vi "sParseRad7String.vi"(0 "Rad7 Input data":string="0501 2.69 \" 2.83 p Sniff\nFRI 21-MAY-99 19:41\n26.8 EC RH: 7% B:7.06V\nTotal Counts: 42.\nLivetime: 27.8min\nA: 0.53\"0.08 cpm 47.3%\nB: 0.02\"0.02 cpm 1.7%\nC: 0.52\"0.08 cpm 46.4%\nD: 0.01\"0.02 cpm 0.9%\nO: 0.04\"0.03 cpm 3.6%") -> (1 "Datanames":string[](array[string]), 2 "Data":dbl[](array[numeric]))   [LabVIEW 2012]
panel:
  out "substring before match":string
  out "array 2":string[][](array[string])
  out "Array":dbl[](array[numeric])
  out "appended array":string[](array[string])
  out "array":string[][](array[string])
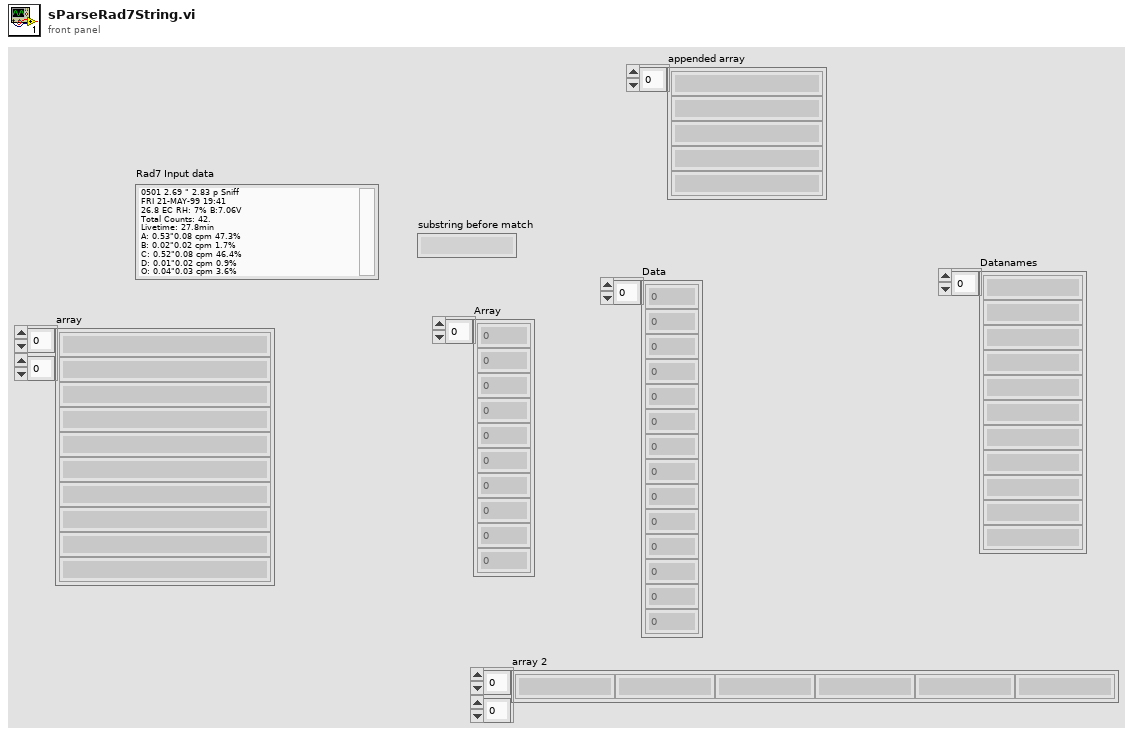
[diagram p1: front panel]
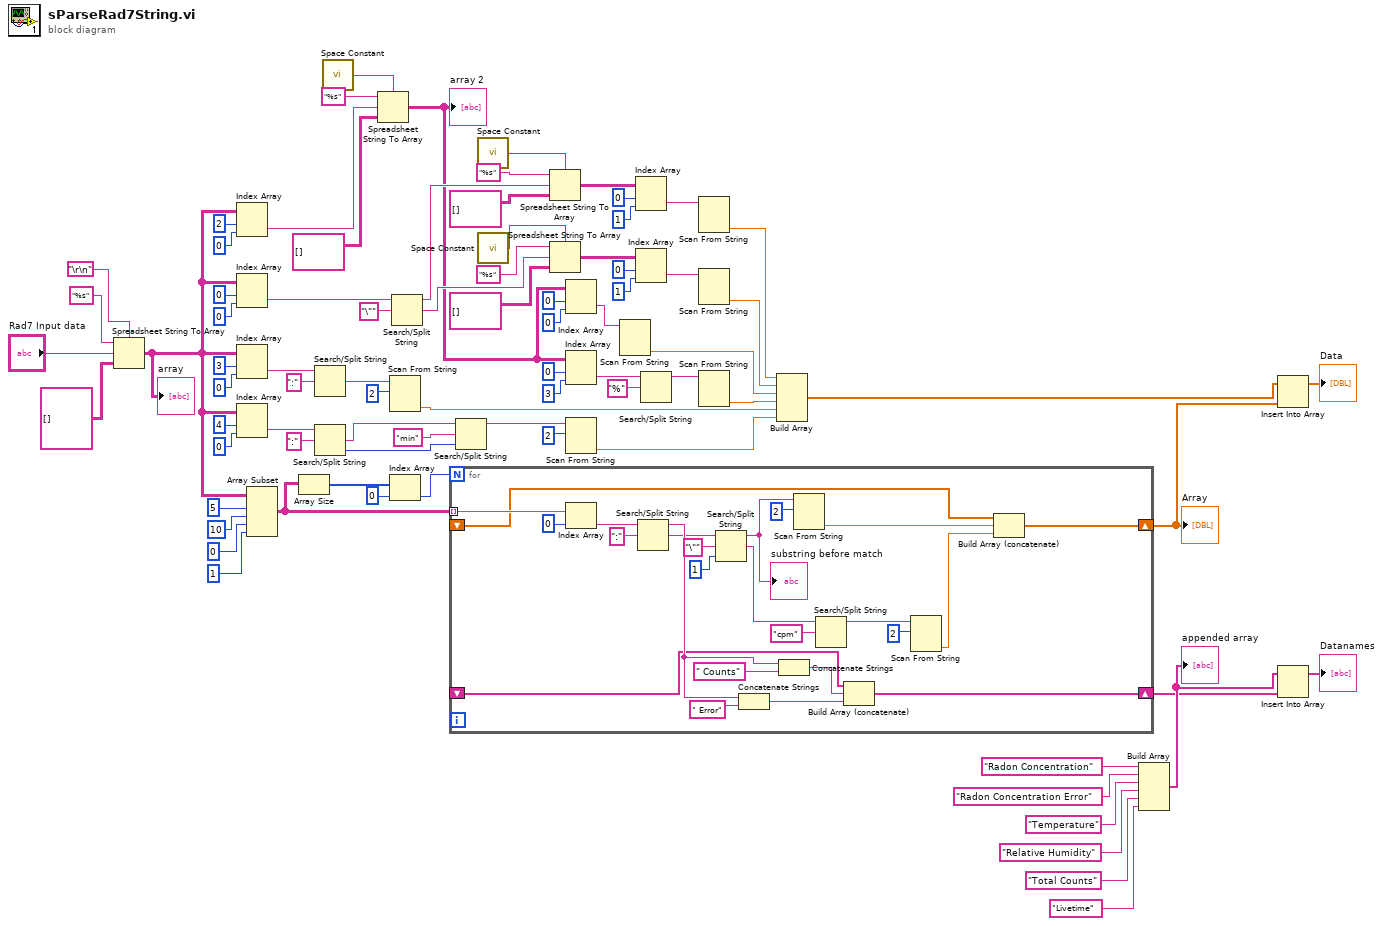
[diagram p0: block diagram]
diagram:
  n1 = Spreadsheet String To Array(delimiter (Tab)="\r\n", format string="%s", spreadsheet string="Rad7 Input data", array type (2D Dbl)=string[][] []) -> (array=w6:string[][])
  "array" <- w6
  n2 = Index Array(array=w6, index (row)=2, index (col)=0) -> (element=w39:string)
  n3 = Index Array(array=w6, index (row)=0, index (col)=0 ("disabled index (col)")) -> (element=w70:string)
  n4 = Index Array(array=w6, index (row)=3, index (col)=0) -> (element=w5:string)
  n5 = Index Array(array=w6, index (row)=4, index (col)=0) -> (element=w18:string)
  n6 = Array Subset(array=w6, index (row)=5 ("index"), length (row)=10 ("length"), index (col)=0 ("index"), length (col)=1 ("length")) -> (w48:string[][])
  n7 = Array Size(array=w48) -> (size(s)=w51:i32[])
  n8 = Search/Split String(string=w5, search string/char (-)=":") -> (match + rest of string=w3:string)  [unwired: 1 in, 2 out]
  n9 = Search/Split String(string=w18, search string/char (-)=":") -> (match + rest of string=w16:string, offset of match=w14:i32)  [unwired: 1 in, 1 out]
  n10 = call <vilib>:"Space Constant.vi"() -> ("String"=w42:string)
  n11 = Spreadsheet String To Array(delimiter (Tab)=w42, format string="%s", spreadsheet string=w39, array type (2D Dbl)=string[][] []) -> (array=w23:string[][])
  "array 2" <- w23
  n12 = Scan From String(input string=w3, initial scan location=u32 2) -> (output 1=w1:dbl)  [unwired: 3 in, 3 out]
  n13 = Index Array(array=w51, index=0) -> (element=w49:i32)
  n14 = Search/Split String(string=w70, search string/char (-)="\"") -> (substring before match=w69:string, match + rest of string=w62:string)  [unwired: 1 in, 1 out]
  n15 = for {
    N: w49 -> [_]
    tunnel: w48 -> [w105] mode=indexing
    shift-right: [w96] -> w30
    shift-left: _ -> [w95]
    shift-right: [w88] -> w27
    shift-left: _ -> [w87]
    n16 = Index Array(array=w105, index=0) -> (element=w102:string)
    n17 = Search/Split String(string=w102, search string/char (-)=":") -> (substring before match=w99:string, match + rest of string=w93:string)  [unwired: 1 in, 1 out]
    n18 = Search/Split String(string=w93, search string/char (-)="\"", offset (0)=1) -> (substring before match=w91:string, match + rest of string=w86:string)  [unwired: 1 out]
    "substring before match" <- w91
    n19 = Concatenate Strings(w99, " Error" ("string")) -> (w97:string)
    n20 = Concatenate Strings(w99, " Counts" ("string")) -> (w98:string)
    n21 = Scan From String(input string=w91, initial scan location=u32 2) -> (output 1=w90:dbl)  [unwired: 3 in, 3 out]
    n22 = Search/Split String(string=w86, search string/char (-)="cpm") -> (substring before match=w84:string)  [unwired: 1 in, 2 out]
    n23 = Build Array (concatenate)(w95, w98, w97) -> (w96:string[])
    n24 = Scan From String(input string=w84, initial scan location=u32 2) -> (output 1=w89:dbl)  [unwired: 3 in, 3 out]
    n25 = Build Array (concatenate)(w87, w90, w89) -> (w88:dbl[])
  }
  "Array" <- w27
  n26 = Search/Split String(string=w16, search string/char (-)="min", offset (0)=w14) -> (substring before match=w13:string)  [unwired: 2 out]
  n27 = call <vilib>:"Space Constant.vi"() -> ("String"=w68:string)
  n28 = call <vilib>:"Space Constant.vi"() -> ("String"=w65:string)
  n29 = Spreadsheet String To Array(delimiter (Tab)=w68, format string="%s", spreadsheet string=w69, array type (2D Dbl)=string[][] []) -> (array=w61:string[][])
  n30 = Spreadsheet String To Array(delimiter (Tab)=w65, format string="%s", spreadsheet string=w62, array type (2D Dbl)=string[][] []) -> (array=w47:string[][])
  n31 = Index Array(array=w23, index (row)=0, index (col)=0 ("disabled index (col)")) -> (element=w33:string)
  n32 = Index Array(array=w23, index (row)=0, index (col)=3 ("disabled index (col)")) -> (element=w22:string)
  n33 = Scan From String(input string=w13, initial scan location=u32 2) -> (output 1=w9:dbl)  [unwired: 3 in, 3 out]
  n34 = Scan From String(input string=w33) -> (output 1=w32:dbl)  [unwired: 4 in, 3 out]
  n35 = Index Array(array=w61, index (row)=0, index (col)=1 ("disabled index (col)")) -> (element=w58:string)
  n36 = Index Array(array=w47, index (row)=0, index (col)=1 ("disabled index (col)")) -> (element=w35:string)
  n37 = Search/Split String(string=w22, search string/char (-)="%") -> (substring before match=w20:string)  [unwired: 1 in, 2 out]
  n38 = Scan From String(input string=w58) -> (output 1=w56:dbl)  [unwired: 4 in, 3 out]
  n39 = Scan From String(input string=w35) -> (output 1=w57:dbl)  [unwired: 4 in, 3 out]
  n40 = Scan From String(input string=w20) -> (output 1=w19:dbl)  [unwired: 4 in, 3 out]
  n41 = Build Array(w56, w57, w32, w19, w1, w9) -> (w28:dbl[])
  n42 = Build Array("Radon Concentration", "Radon Concentration Error", "Temperature", "Relative Humidity", "Total Counts", "Livetime") -> (w31:string[])
  "appended array" <- w31
  n43 = Insert Into Array(array=w28, new element=w27) -> (→"Data":dbl[])  [unwired: 1 in]
  n44 = Insert Into Array(array=w31, new element=w30) -> (→"Datanames":string[])  [unwired: 1 in]
